vi "Write Icon.lvclass.vi"(8 "error in (no error)":errorcluster, 10 "Icon.lvclass":refnum<class "Icon.lvclass">, 11 "NotifyIcon in":refnum<class "NotifyIcon.lvclass">) -> (0 "error out":errorcluster, 3 "NotifyIcon out":refnum<class "NotifyIcon.lvclass">)   [LabVIEW 2016, in "NotifyIcon.lvclass"]
uses:
  NotifyIcon.lvclass
  Icon/Icon.lvclass
  NotifyIcon.lvclass/NotifyIcon.ctl
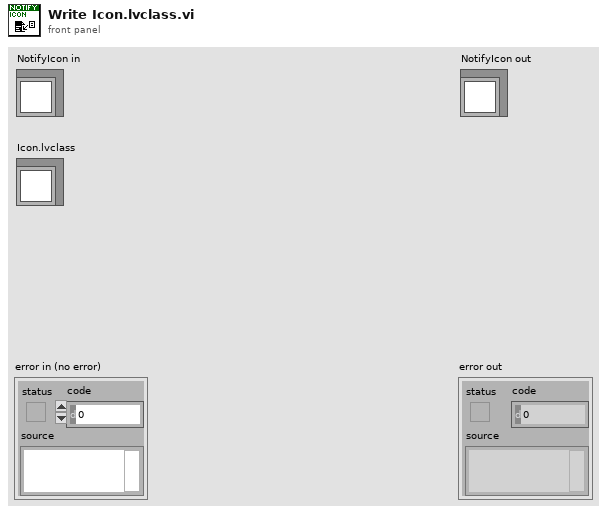
[diagram p1: front panel]
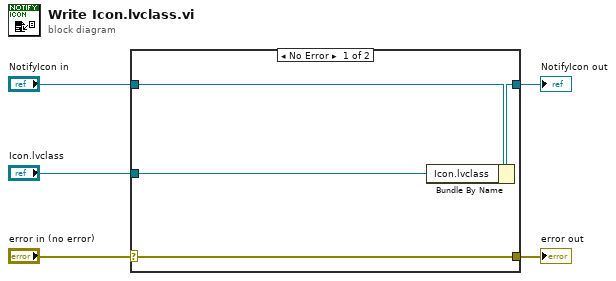
[diagram p0: block diagram]
diagram:
  n1 = case shown="No Error" "error in (no error)" {
    selector: "error in (no error)" -> [w9 w10]
    tunnel: [w9 w10] -> w4
    tunnel: [w7 w11] -> w2
    tunnel: "NotifyIcon in" -> [w8 w11]
    tunnel: "Icon.lvclass" -> [w6 _]
    frame No Error {
      n2 = Bundle By Name(cluster=w8, "Icon.lvclass"=w6) -> (w7:refnum<class "NotifyIcon.lvclass">)
    }
    frame Error {
    }
  }
  "error out" <- w4
  "NotifyIcon out" <- w2
